vi "2d to 1D.vi"() -> ()   [LabVIEW 2014]
panel:
  out "transposed array":dbl[][](array[numeric])
  out "output array":dbl[](array[numeric])
  out "unsigned byte array":u8[](array[numeric])
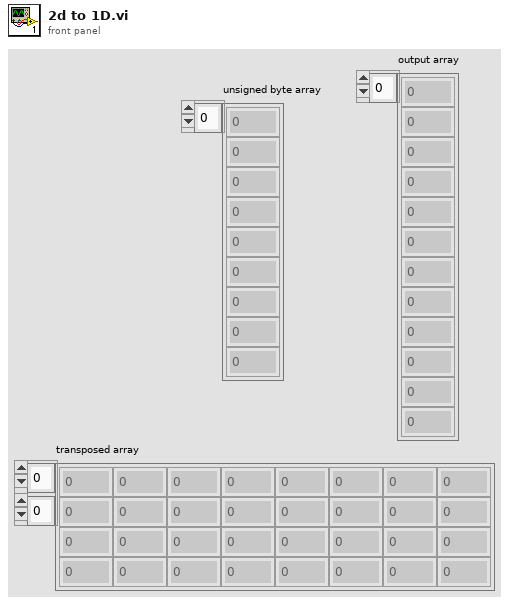
[diagram p1: front panel]
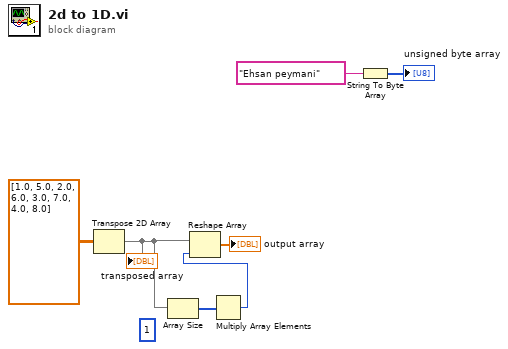
[diagram p0: block diagram]
diagram:
  (unwired) 1 ("dimension size")
  n1 = Transpose 2D Array(2D array=dbl[][] [[1.0, 5.0], [2.0, 6.0], [3.0, 7.0], [4.0, 8.0]]) -> (transposed array=w1:dbl[][])
  "transposed array" <- w1
  n2 = Array Size(array=w1) -> (size(s)=w4:i32[])
  n3 = Multiply Array Elements(1:w4) -> (0:w3:i32)
  n4 = Reshape Array(w1, w3) -> (→"output array":dbl[])
  n5 = String To Byte Array(string="Ehsan peymani") -> (unsigned byte array=→"unsigned byte array":u8[])
